vi "SCP_read_VS.vi"(8 "error_in":errorcluster, 10 "Ref":T2, 11 "Compiled.Settings":T3={"Name"="", "RDB Data Receive "=[], "RDB Data Sent"=[], "vclient"=path "", "Network Settings"={"IP adress"="127.0.0.1", "RDB"={"Protocol"=enum."TCP", "Tx Port"=10, "Rx Port"=10, "Buffer Size"=204800, "Timeout"=10}, "SCP"={"Protocol"=enum."UDP", "Tx Port"=48190, "Rx Port"=48190, "Buffer Size"=204800, "Timeout"=10}}, "SensorInfos"=[], "mmanager"=path "", "Scenario Paths"=[], "Custom SCP Commands"=[]}) -> (0 "error_out":errorcluster, 1 "SCP_Cluster_out":T1)   [LabVIEW 2020, in "Vires VTD Engine.lvlib"]
uses:
  Vires VTD Engine.lvlib
  Shared/Compiled.Settings.ctl
  System Explorer/RDB Data.ctl
  RDB/RDB Object.ctl
  RDB/RDB Player Object.ctl
  Shared/Network Settings.ctl
  Shared/Protocol.ctl
  Shared/SensorInfos.ctl
  Shared/SensorInfo.ctl
  Shared/Sensor Name.ctl
  MM/MM Data.ctl
  MM/MM Objects.ctl
  MM/MM Object.ctl
  <vilib>/NI/NIVS Inline Async API/_Data Access Engine/Data Access Engine/Types/ReadWrite.DVR.ctl
  <vilib>/NI/NIVS Inline Async API/_Data Access Engine/Access Type Classes/ReadWrite/ReadWrite.lvclass
  Type/SCP_Cluster.ctl
  <vilib>/NI/NIVS Inline Async API/_Data Access Engine/Access Type Classes/ReadWrite/ReadWrite.lvclass/ReadWrite.ctl
  <vilib>/NI/NIVS Inline Async API/_Data Access Engine/Data Access Engine/Methods/ReadWrite.Data.Read.vi
  <vilib>/NI/NIVS Inline Async API/_Data Access Engine/Access Type Classes/ReadWrite/ReadWrite.ProcessData.Read.vi
  <vilib>/NI/NIVS Inline Async API/_Data Access Engine/Data Access Engine/Data Access Engine.lvclass
  SCP/SCP.lvlib
  RDB/RDB.lvlib
  Shared/Vires VTD Shared.lvlib
  MM/MM.lvlib
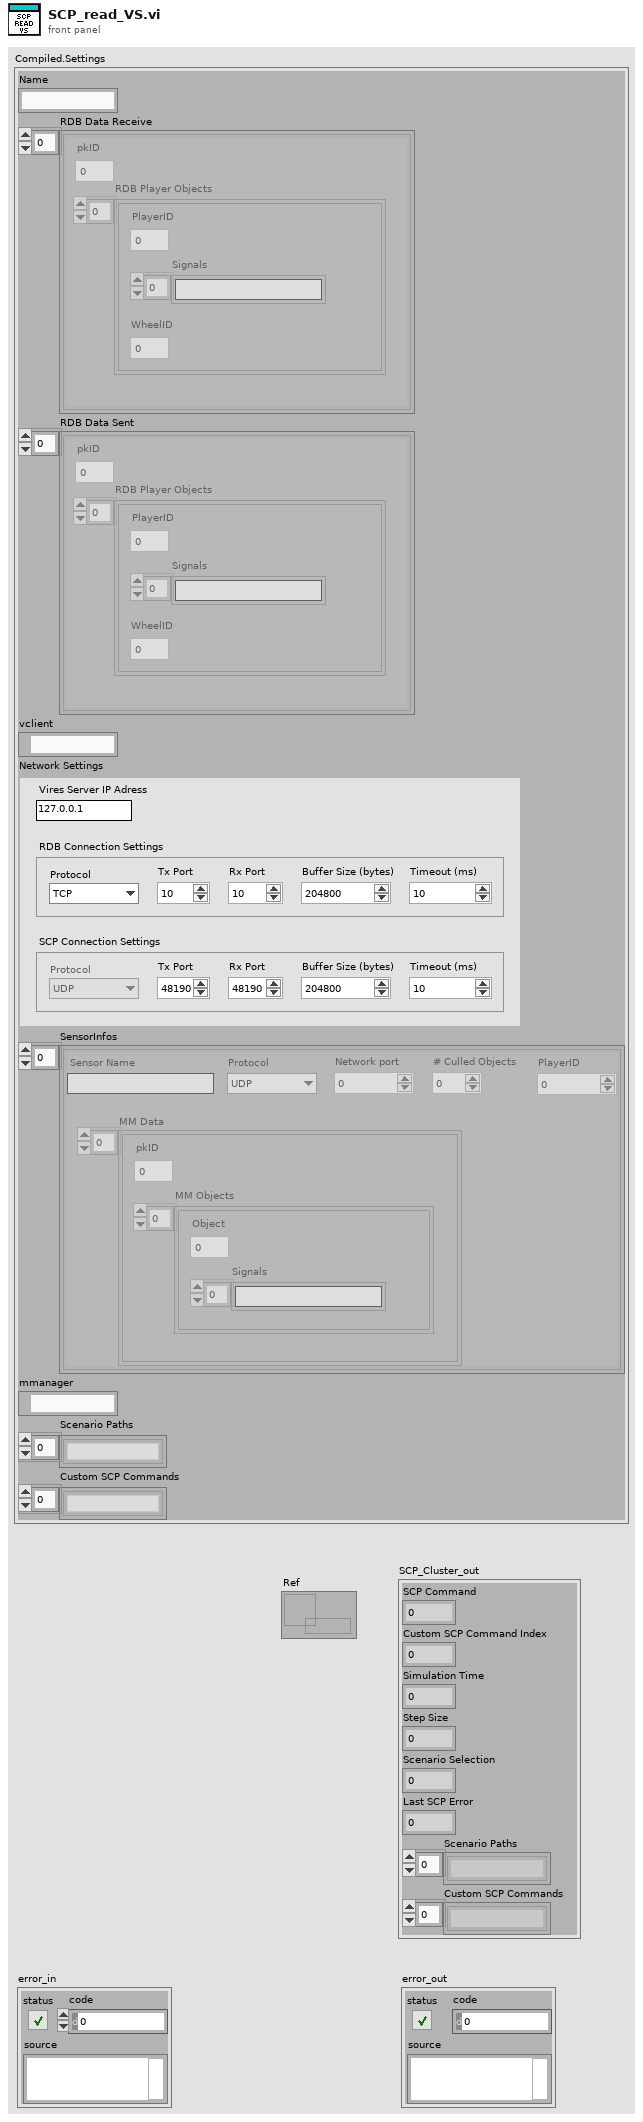
[diagram p1: front panel]
types:
  T1 = typedef "SCP.lvlib/SCP_Cluster.ctl" = cluster{"SCP Command ":i32, "Custom SCP Command Index":i32, "Simulation Time":i32, "Step Size":i32, "Scenario Selection":i32, "Last SCP Error":i32, "Scenario Paths":string[], "Custom SCP Commands":string[]}
  T2 = typedef "Data Access Engine.lvlib/Data Access Engine.lvclass/ReadWrite.DVR.ctl" = refnum<data-value>
  T3 = typedef "Vires VTD Shared.lvlib/Compiled.Settings.ctl" = cluster{"Name":string, "RDB Data Receive ":T4, "RDB Data Sent":T4, "vclient":path, "Network Settings":T7, "SensorInfos":T9, "mmanager":path, "Scenario Paths":string[], "Custom SCP Commands":string[]}
  T4 = typedef "Vires VTD Shared.lvlib/RDB Data.ctl" = T5[]
  T5 = typedef "RDB.lvlib/RDB Object.ctl" = cluster{"pkID":i32, "RDB Player Objects":T6[]}
  T6 = typedef "RDB.lvlib/RDB Player Object.ctl" = cluster{"PlayerID":i32, "Signals":string[], "WheelID":i32}
  T7 = typedef "Vires VTD Shared.lvlib/Network Settings.ctl" = cluster{"IP adress":string, "RDB":cluster{"Protocol":T8, "Tx Port":u16, "Rx Port":u16, "Buffer Size":i32, "Timeout":u16}, "SCP":cluster{"Protocol":T8, "Tx Port":u16, "Rx Port":u16, "Buffer Size":i32, "Timeout":u16}}
  T8 = typedef "Vires VTD Shared.lvlib/Protocol.ctl" = enum16{"UDP", "TCP"}
  T9 = typedef "Vires VTD Shared.lvlib/SensorInfos.ctl" = T10[]
  T10 = typedef "Vires VTD Shared.lvlib/SensorInfo.ctl" = cluster{"Sensor Name":T11, "Protocol":T8, "Network port":i32, "# Culled Objects":i32, "PlayerID":u8, "MM Data":T12}
  T11 = typedef "Vires VTD Shared.lvlib/Sensor Name.ctl" = string
  T12 = typedef "Vires VTD Shared.lvlib/MM Data.ctl" = T13[]
  T13 = typedef "MM.lvlib/MM Objects.ctl" = cluster{"pkID":i32, "MM Objects":T14[]}
  T14 = typedef "MM.lvlib/MM Object.ctl" = cluster{"Object":i32, "Signals":string[]}
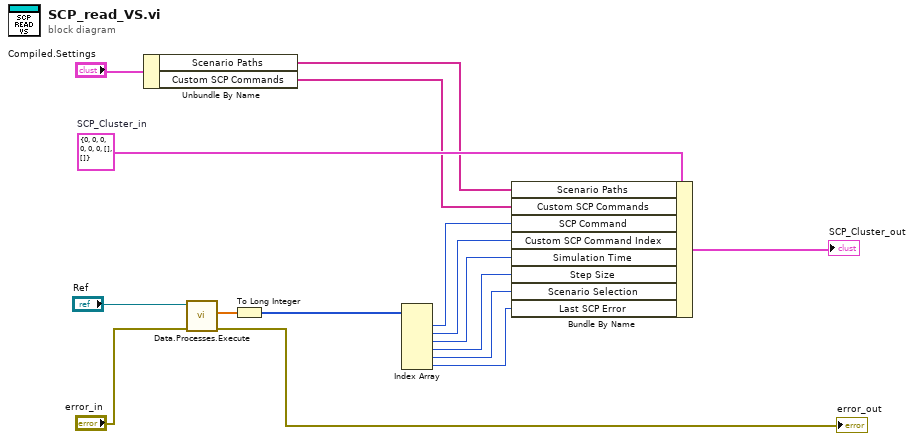
[diagram p0: block diagram]
diagram:
  w13 = T1 {"SCP Command "=0, "Custom SCP Command Index"=0, "Simulation Time"=0, "Step Size"=0, "Scenario Selection"=0, "Last SCP Error"=0, "Scenario Paths"=[], "Custom SCP Commands"=[]}  # SCP_Cluster_in
  n1 = Unbundle By Name("Compiled.Settings") -> ("Scenario Paths"=w12:string[], "Custom SCP Commands"=w11:string[])
  n2 = call-poly <vilib>:"Data.Processes.Execute.vi"("error in (no error)"="error_in", "Ref"="Ref") -> ("error out"=→"error_out":errorcluster, "Data"=w10:dbl[])  [unwired: 6 in, 2 out]
  n3 = To Long Integer(number=w10) -> (32bit integer=w7:i32[])
  n4 = Index Array(array=w7) -> (element #1=w6:i32, element #2=w5:i32, element #3=w4:i32, element #4=w3:i32, element #5=w2:i32, element #6=w1:i32)  [unwired: 6 in]
  n5 = Bundle By Name(cluster=w13, "Scenario Paths"=w12, "Custom SCP Commands"=w11, "SCP Command"=w6, "Custom SCP Command Index"=w5, "Simulation Time"=w4, "Step Size"=w3, "Scenario Selection"=w2, "Last SCP Error"=w1) -> (→"SCP_Cluster_out":T1)
